vi "udp write.vi"(5 "UDP Port":u16, 7 "UDP IP Address":string, 8 "error in (no error)":errorcluster, 10 "Data Array of Clusters (in)":cluster{"Data Array":string[], "Numeric":i32}[](array[cluster]), 11 "UDP ID (in)":refnum<k16>) -> (0 "error out":errorcluster, 2 "Data Array of Cluster (out)":cluster{"Data Array":string[], "Numeric":i32}[](array[cluster]), 3 "UDP ID (out)":refnum<k16>)   [LabVIEW 2021]
panel:
  out "deleted portion":string[](array[string])
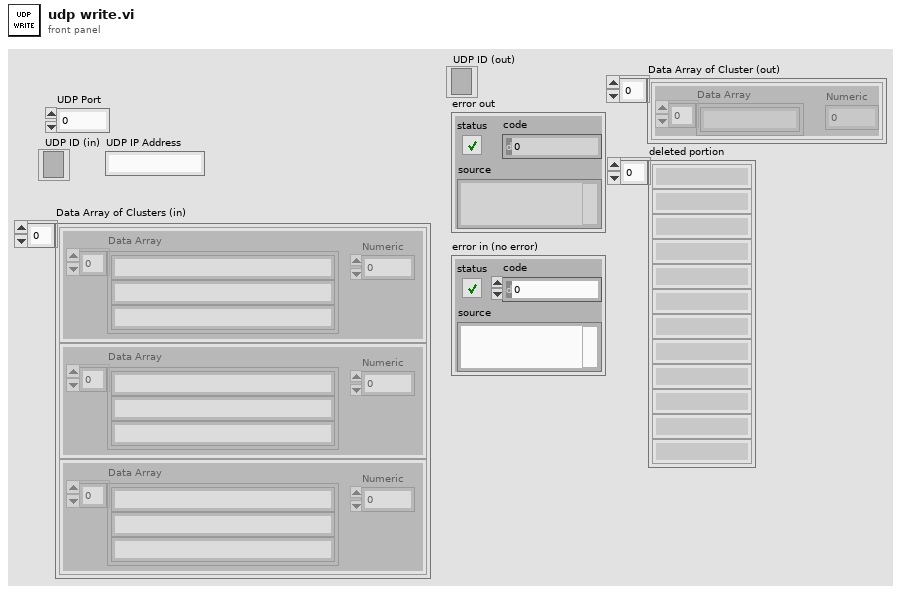
[diagram p1: front panel]
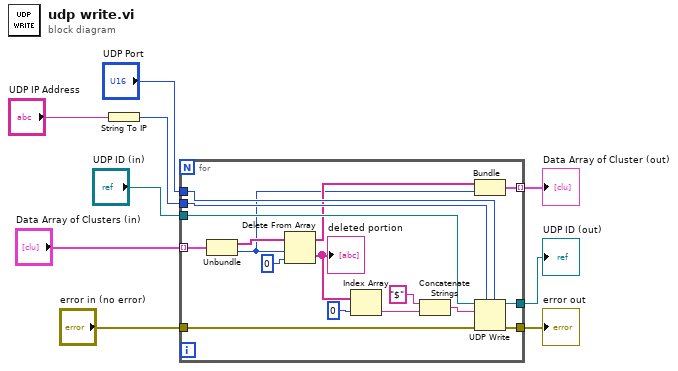
[diagram p0: block diagram]
diagram:
  n1 = String To IP(1:"UDP IP Address") -> (0:w2:u32)
  n2 = for {
    tunnel: w2 -> [w26]
    tunnel: "UDP Port" -> [w25]
    tunnel: "Data Array of Clusters (in)" -> [w11] mode=indexing
    tunnel: "error in (no error)" -> [w21]
    tunnel: "UDP ID (in)" -> [w24]
    tunnel: [w23] -> w6
    tunnel: [w22] -> w5
    tunnel: [w17] -> w3 mode=indexing
    n3 = Unbundle(w11) -> ("Data Array"=w20:string[], "Numeric"=w10:i32)
    n4 = Delete From Array(array=w20, length=w10, index=0) -> (deleted portion=w16:string[], array with subset deleted=w18:string[])
    "deleted portion" <- w16
    n5 = Index Array(array=w16, index=0) -> (element=w14:string)
    n6 = Concatenate Strings("$" ("string"), w14) -> (w13:string)
    n7 = Bundle("Data Array"=w18, "Numeric"=w10) -> (w17:cluster{"Data Array":string[], "Numeric":i32})  [unwired: 1 in]
    n8 = UDP Write(address=w26, port or service name=w25, connection ID=w24, data in=w13, 8:w21) -> (error out=w22:errorcluster, 3:w23:refnum<k16>)  [unwired: 1 in]
  }
  "UDP ID (out)" <- w6
  "error out" <- w5
  "Data Array of Cluster (out)" <- w3
